vi "HOST_0505_2518.vi"() -> ()   [LabVIEW 2018]
uses:
  <vilib>/userdefined/High Color/nirio_resource_hc.ctl
  <instrlib>/niDCPower/nidcpower.llb/niDCPower Measurement Type.ctl
  <vilib>/FPGAPlugInAG/PXI-7953R/niLvFpga_Open_PXI-7953R.vi
  <vilib>/rvi/interface/common/dynamic/niFpgaDynamicAddResources.vi
  <vilib>/FPGAPlugInAG/Dynamic/niLvFpga_Reset_Dynamic.vi
  <vilib>/FPGAPlugInAG/Dynamic/niLvFpga_Run_Dynamic.vi
  <vilib>/Utility/error.llb/Error Cluster From Error Code.vi
  <vilib>/rvi/errors/niLvFpgaAdjustHostInterfaceError.vi
  <vilib>/FPGAPlugInAG/Dynamic/niLvFpga_Close_Dynamic.vi
  <vilib>/rvi/interface/nirviOpenFPGA/nirviOpenFPGA.xnode
  GSENSE2020BSI/FPGA Bitfiles/GSENSE2020_FPGATarget_Target_dmqGfihq6bQ.lvbitx
  <vilib>/rvi/interface/nirviMethod/nirviMethod.xnode
  <vilib>/rvi/interface/nirviReadWriteControl/nirviReadWriteControl.xnode
  <vilib>/rvi/interface/nirviCloseFPGA/nirviCloseFPGA.xnode
  NiFpgaLv.dll
  <vilib>/rvi/interface/Simulation/niFpgaSimulationCallBeginRW.vi
panel:
  out "SPI_OUT":bool[](array[boolean])
  in  "Запись":bool[](array[boolean])=[TRUE, TRUE, FALSE, FALSE, FALSE, FALSE, FALSE, FALSE, TRUE, FALSE, TRUE, FALSE, TRUE, TRUE, TRUE, FALSE, FALSE, TRUE, FALSE, FALSE, TRUE, TRUE, FALSE, FALSE, TRUE, TRUE, FALSE, TRUE, TRUE, TRUE, FALSE, FALSE, FALSE, TRUE, TRUE, FALSE, FALSE, TRUE, TRUE, TRUE, TRUE, FALSE, FALSE, TRUE, FALSE, TRUE, FALSE, FALSE, FALSE, TRUE, FALSE, TRUE, TRUE, FALSE, TRUE, TRUE, TRUE, TRUE, TRUE, FALSE, TRUE, TRUE, TRUE, FALSE, TRUE, FALSE, FALSE, FALSE, TRUE, TRUE, TRUE, FALSE, FALSE, FALSE, FALSE, FALSE, FALSE, FALSE, FALSE, FALSE, FALSE, FALSE, FALSE, FALSE, FALSE, FALSE, TRUE, TRUE, TRUE, TRUE, FALSE, FALSE, FALSE, FALSE, FALSE, TRUE, TRUE, FALSE, TRUE, FALSE, TRUE, FALSE, FALSE, FALSE, FALSE, TRUE, FALSE, FALSE, FALSE, TRUE, TRUE, FALSE, TRUE, FALSE, FALSE, FALSE, TRUE, TRUE, TRUE, TRUE, TRUE, FALSE, FALSE, TRUE, FALSE, FALSE, FALSE, TRUE, TRUE, FALSE, TRUE, FALSE, FALSE, TRUE, TRUE, TRUE, TRUE, TRUE, TRUE, FALSE, FALSE, TRUE, TRUE, FALSE, FALSE, TRUE, TRUE, TRUE, TRUE, FALSE, FALSE, TRUE, TRUE, FALSE, FALSE, FALSE, FALSE, FALSE, TRUE, TRUE, FALSE, FALSE, TRUE, FALSE, FALSE, FALSE, FALSE, FALSE, FALSE, FALSE, FALSE, FALSE, FALSE, FALSE, FALSE, FALSE, FALSE, FALSE, FALSE, FALSE, TRUE, FALSE, FALSE, FALSE, FALSE, FALSE, FALSE, FALSE, TRUE, TRUE, FALSE, TRUE, TRUE, TRUE, TRUE, FALSE, TRUE, FALSE, FALSE, FALSE, FALSE, FALSE, FALSE, FALSE, FALSE, FALSE, FALSE, TRUE, TRUE, TRUE, TRUE, TRUE, TRUE, TRUE, TRUE, FALSE, FALSE, TRUE, TRUE, FALSE, FALSE, TRUE, TRUE, TRUE, TRUE, TRUE, TRUE, TRUE, FALSE, FALSE, FALSE, FALSE, TRUE, TRUE, TRUE, FALSE, TRUE, TRUE, FALSE, TRUE, FALSE, TRUE, FALSE, FALSE, FALSE, FALSE, FALSE, FALSE, FALSE, TRUE, TRUE, TRUE, FALSE, TRUE, TRUE, FALSE]
  in  "3,3V_LVDS, V":dbl caption="voltage level" format="%_6p"
  in  "3,3V_LVDS_curlim":dbl=0.1 caption="current limit" format="%_6p"
  out "3,3V_LVDS_char":dbl(graph)=1.5967060684808935e-06
  in  "VDDPIX, V":dbl caption="voltage level" format="%_6p"
  in  "VDDPIX_curlim":dbl=0.1 caption="current limit" format="%_6p"
  out "VDDPIX_char":dbl(graph)=1.5967060684808935e-06
  in  "VG_RSTH, V":dbl caption="voltage level" format="%_6p"
  in  "VG_RSTH_curlim":dbl=0.1 caption="current limit" format="%_6p"
  out "VG_RSTH_char":dbl(graph)=1.5967060684808935e-06
  in  "LED, V":dbl caption="voltage level" format="%_6p"
  in  "LED_curlim":dbl=0.1 caption="current limit" format="%_6p"
  out "LED_char":dbl(graph)=1.5967060684808935e-06
  in  "VDD33A, V":dbl caption="voltage level" format="%_6p"
  in  "VDD33A_curlim":dbl=0.1 caption="current limit" format="%_6p"
  out "VDD33A_char":dbl(graph)=1.5967060684808935e-06
  in  "W(T)/R(F)":bool
  in  "Автомат":bool
  in  "VTXH, V":dbl caption="voltage level" format="%_6p"
  in  "VDDIO, V":dbl caption="voltage level" format="%_6p"
  in  "VDDCL, V":dbl caption="voltage level" format="%_6p"
  in  "VDD13, V":dbl caption="voltage level" format="%_6p"
  in  "VTXH_curlim":dbl=0.1 caption="current limit" format="%_6p"
  in  "VGRSTL_curlim":dbl=0.1 caption="current limit" format="%_6p"
  in  "VDDIO_curlim":dbl=0.1 caption="current limit" format="%_6p"
  in  "VDDCL_curlim":dbl=0.1 caption="current limit" format="%_6p"
  in  "VTXL_curlim":dbl=0.09 caption="current limit" format="%_6p"
  in  "VDD13_curlim":dbl=0.1 caption="current limit" format="%_6p"
  in  "VGRSTL, V":dbl caption="voltage level" format="%_6p"
  in  "VTXL, V":dbl caption="voltage level" format="%_6p"
  out "VTXH_char":dbl(graph)=-0.007753012065680951
  out "VGRSTL_char":dbl(graph)=6.909391540672134e-05
  out "VDDIO_char":dbl(graph)=9.424895165128459e-05
  out "VDDCL_char":dbl(graph)=-9.950040532110056e-06
  out "VTXL_char":dbl(graph)=9.067752968783287e-05
  out "VDD13_char":dbl(graph)=1.5967060684808935e-06
  in  "VDDPIX_selcur":dbl=0.09 caption="current limit" format="%_6p"
  in  "VDD33A_selcur":dbl=0.09 caption="current limit" format="%_6p"
  in  "VDD13_selcur":dbl=0.09 caption="current limit" format="%_6p"
  in  "VTXL_selcur":dbl=0.1 caption="current limit" format="%_6p"
  out "VDDCL_cur":dbl caption="measurement" format="%_6g"
  out "VTXL_cur":dbl caption="measurement" format="%_6g"
  out "VDD13_cur":dbl caption="measurement" format="%_6g"
  out "VDD33A_cur":dbl caption="measurement" format="%_6g"
  in  "SEL_Time, ms":u32=100
  in  "VG_RSTH_selcur":dbl=0.09 caption="current limit" format="%_6p"
  in  "VTXH_selcur":dbl=0.09 caption="current limit" format="%_6p"
  in  "VGRSTL_selcur":dbl=0.09 caption="current limit" format="%_6p"
  in  "VDDIO_selcur":dbl=0.09000000000000001 caption="current limit" format="%_6p"
  in  "VDDCL_selcur":dbl=0.09 caption="current limit" format="%_6p"
  out "VDDPIX_cur":dbl caption="measurement" format="%_6g"
  out "VDDIO_cur":dbl caption="measurement" format="%_6g"
  out "VGRSTL_cur":dbl caption="measurement" format="%_6g"
  out "VTXH_cur":dbl caption="measurement" format="%_6g"
  out "VG_RSTH_cur":dbl caption="measurement" format="%_6g"
  out "VDDPIX":u16
  out "VDDPIX":bool
  out "VDD33A":u16
  out "VDD33A":bool
  out "VDD13":u16
  out "VDD13":bool
  out "VTXL":u16
  out "VTXL":bool
  in  "3":refnum<k15>="PXI1Slot7" caption="1"
  in  "Проверка сбоев":bool
  out "SEU":bool
  out "SEU":u16
  in  "SPI":bool
  out "REG":bool
  in  "SAVE":bool
  in  "MOVIE":bool
  out "Картинка":bool
  out "Записали FIFO":bool
  in  "Хватит ждать!":bool
  in  "FRAME!":bool
  in  "SYS_RESET_N":bool
  out "SEL":bool
  in  "SIM_SEL":bool
  out "VG_RSTH":u16
  out "VDDCL":u16
  out "VTXH":u16
  out "VDDIO":u16
  out "VGRSTL":u16
  out "VG_RSTH":bool
  out "VDDCL":bool
  out "VTXH":bool
  out "VDDIO":bool
  out "VGRSTL":bool
  in  "Стоп":bool
  in  "Питание":bool
  in  "LED":bool caption="output enabled"
  in  "0":refnum<k15>="PXI1Slot5" caption="1"
  in  "1":refnum<k15>="PXI1Slot6"
  in  "2":refnum<k15>="PXI1Slot7" caption="1"
  in  "resource name 2":T1="PXI1Slot9"
  in  "SEU":path=path "C:/VPL/LabView/GSENSE2020BSI/SEU"
  in  "SEL":path=path "C:/VPL/LabView/GSENSE2020BSI/SEL"
  out "Номер образца":string="1"
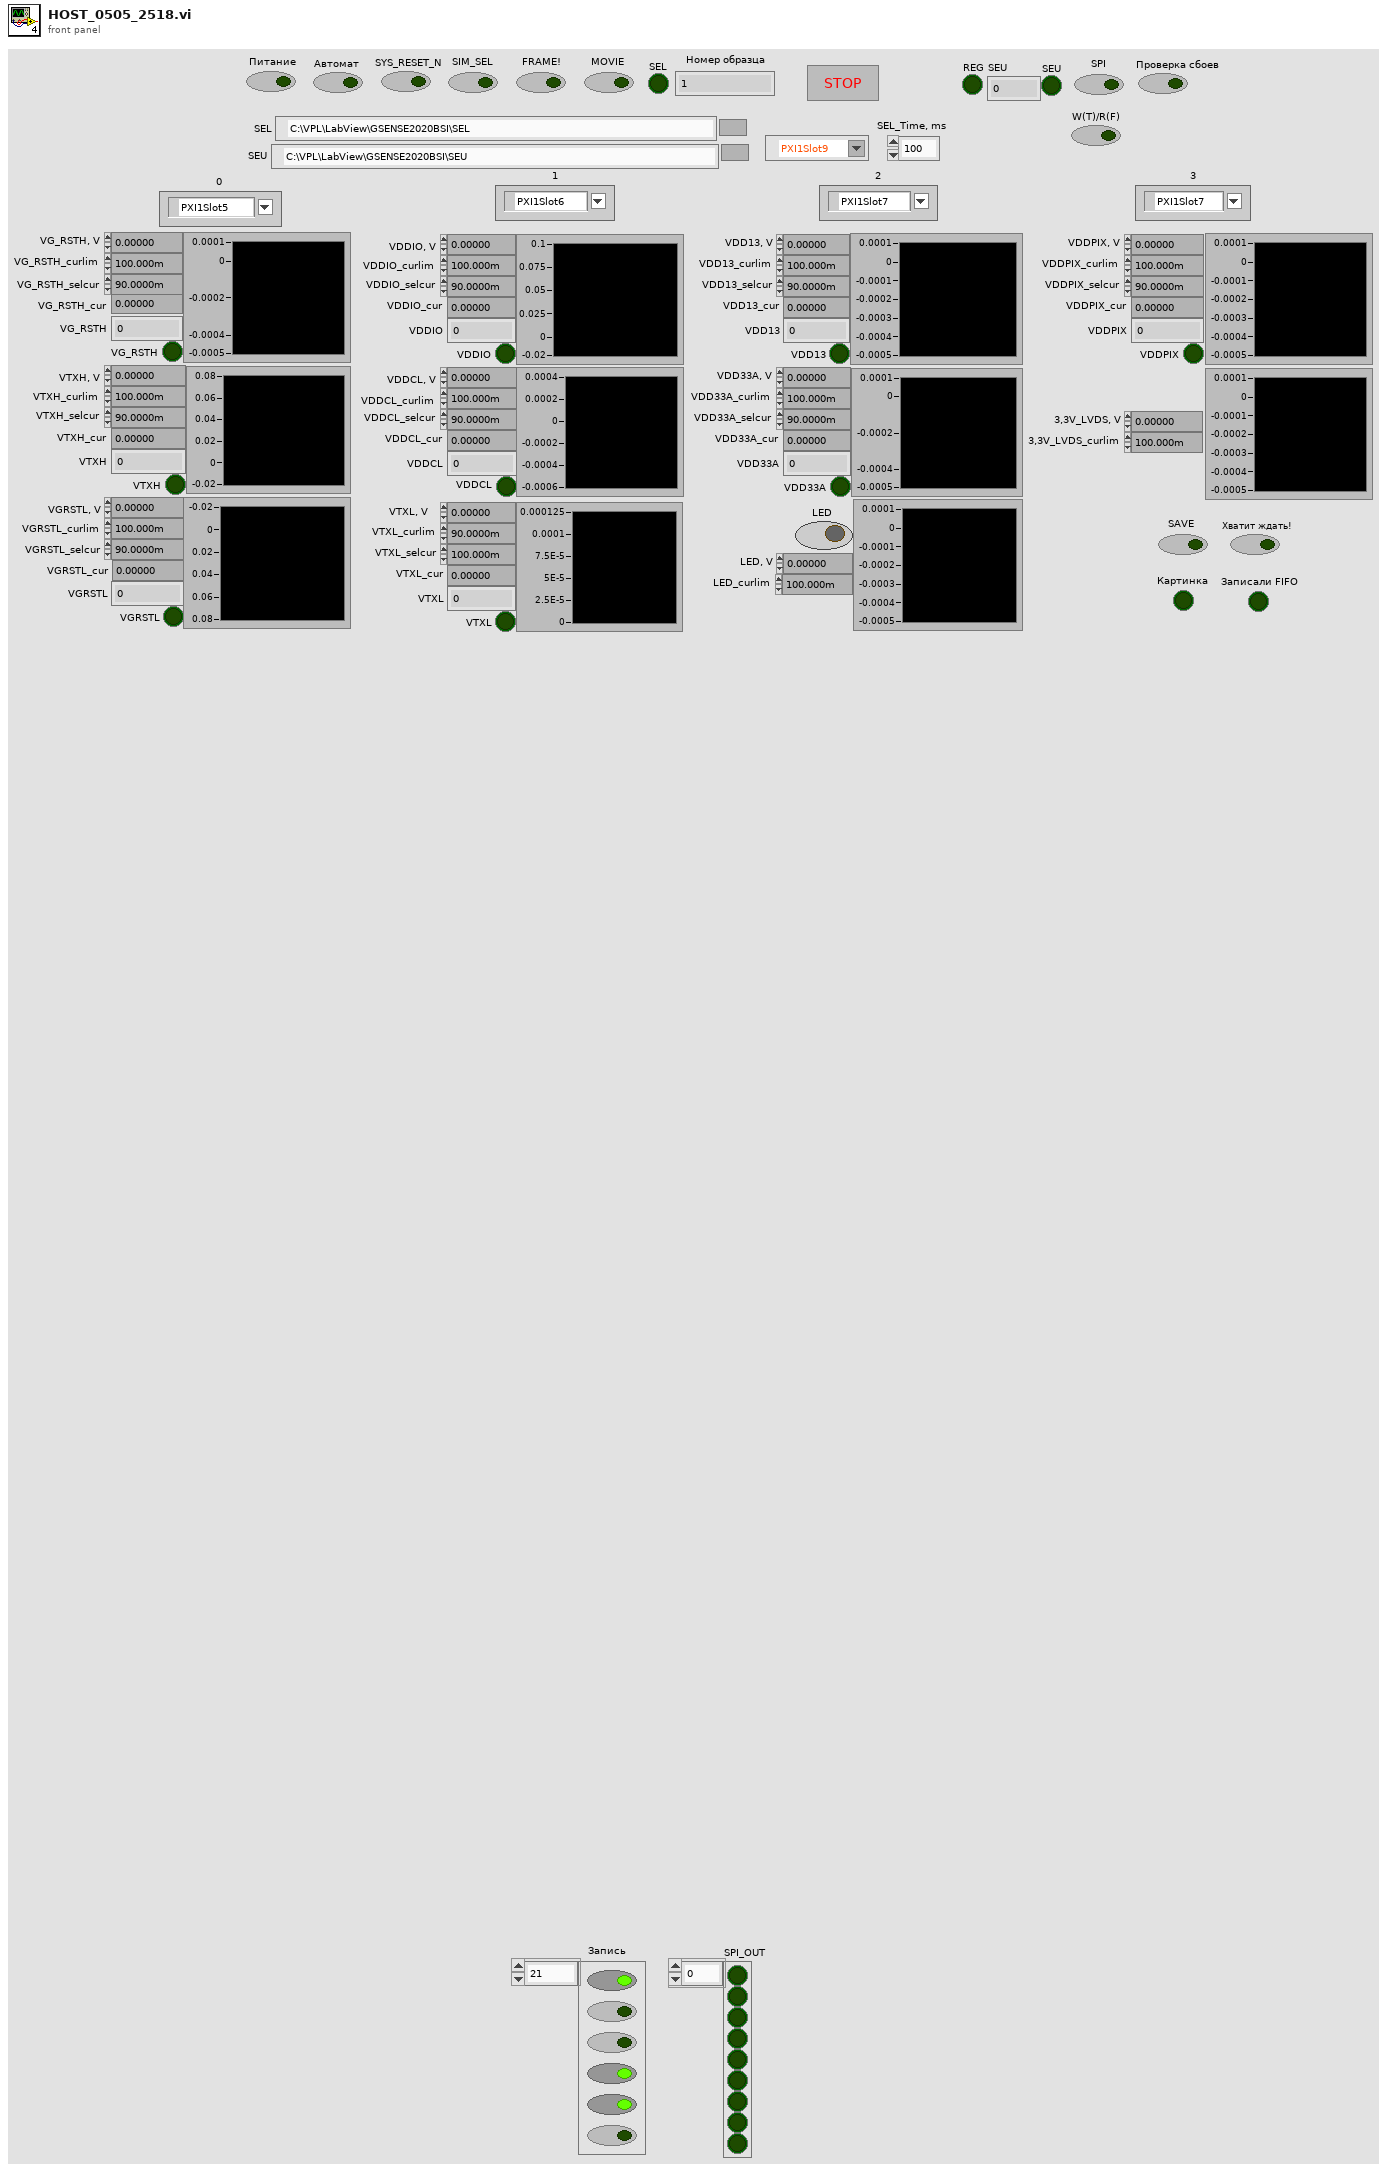
[diagram p1: front panel]
types:
  T1 = typedef "nirio_resource_hc.ctl" = tag
  T2 = enum16{"open", "replace", "create", "open or create", "replace or create", "replace or create with confirmation"}
  T3 = typedef "niDCPower Measurement Type.ctl" = i32
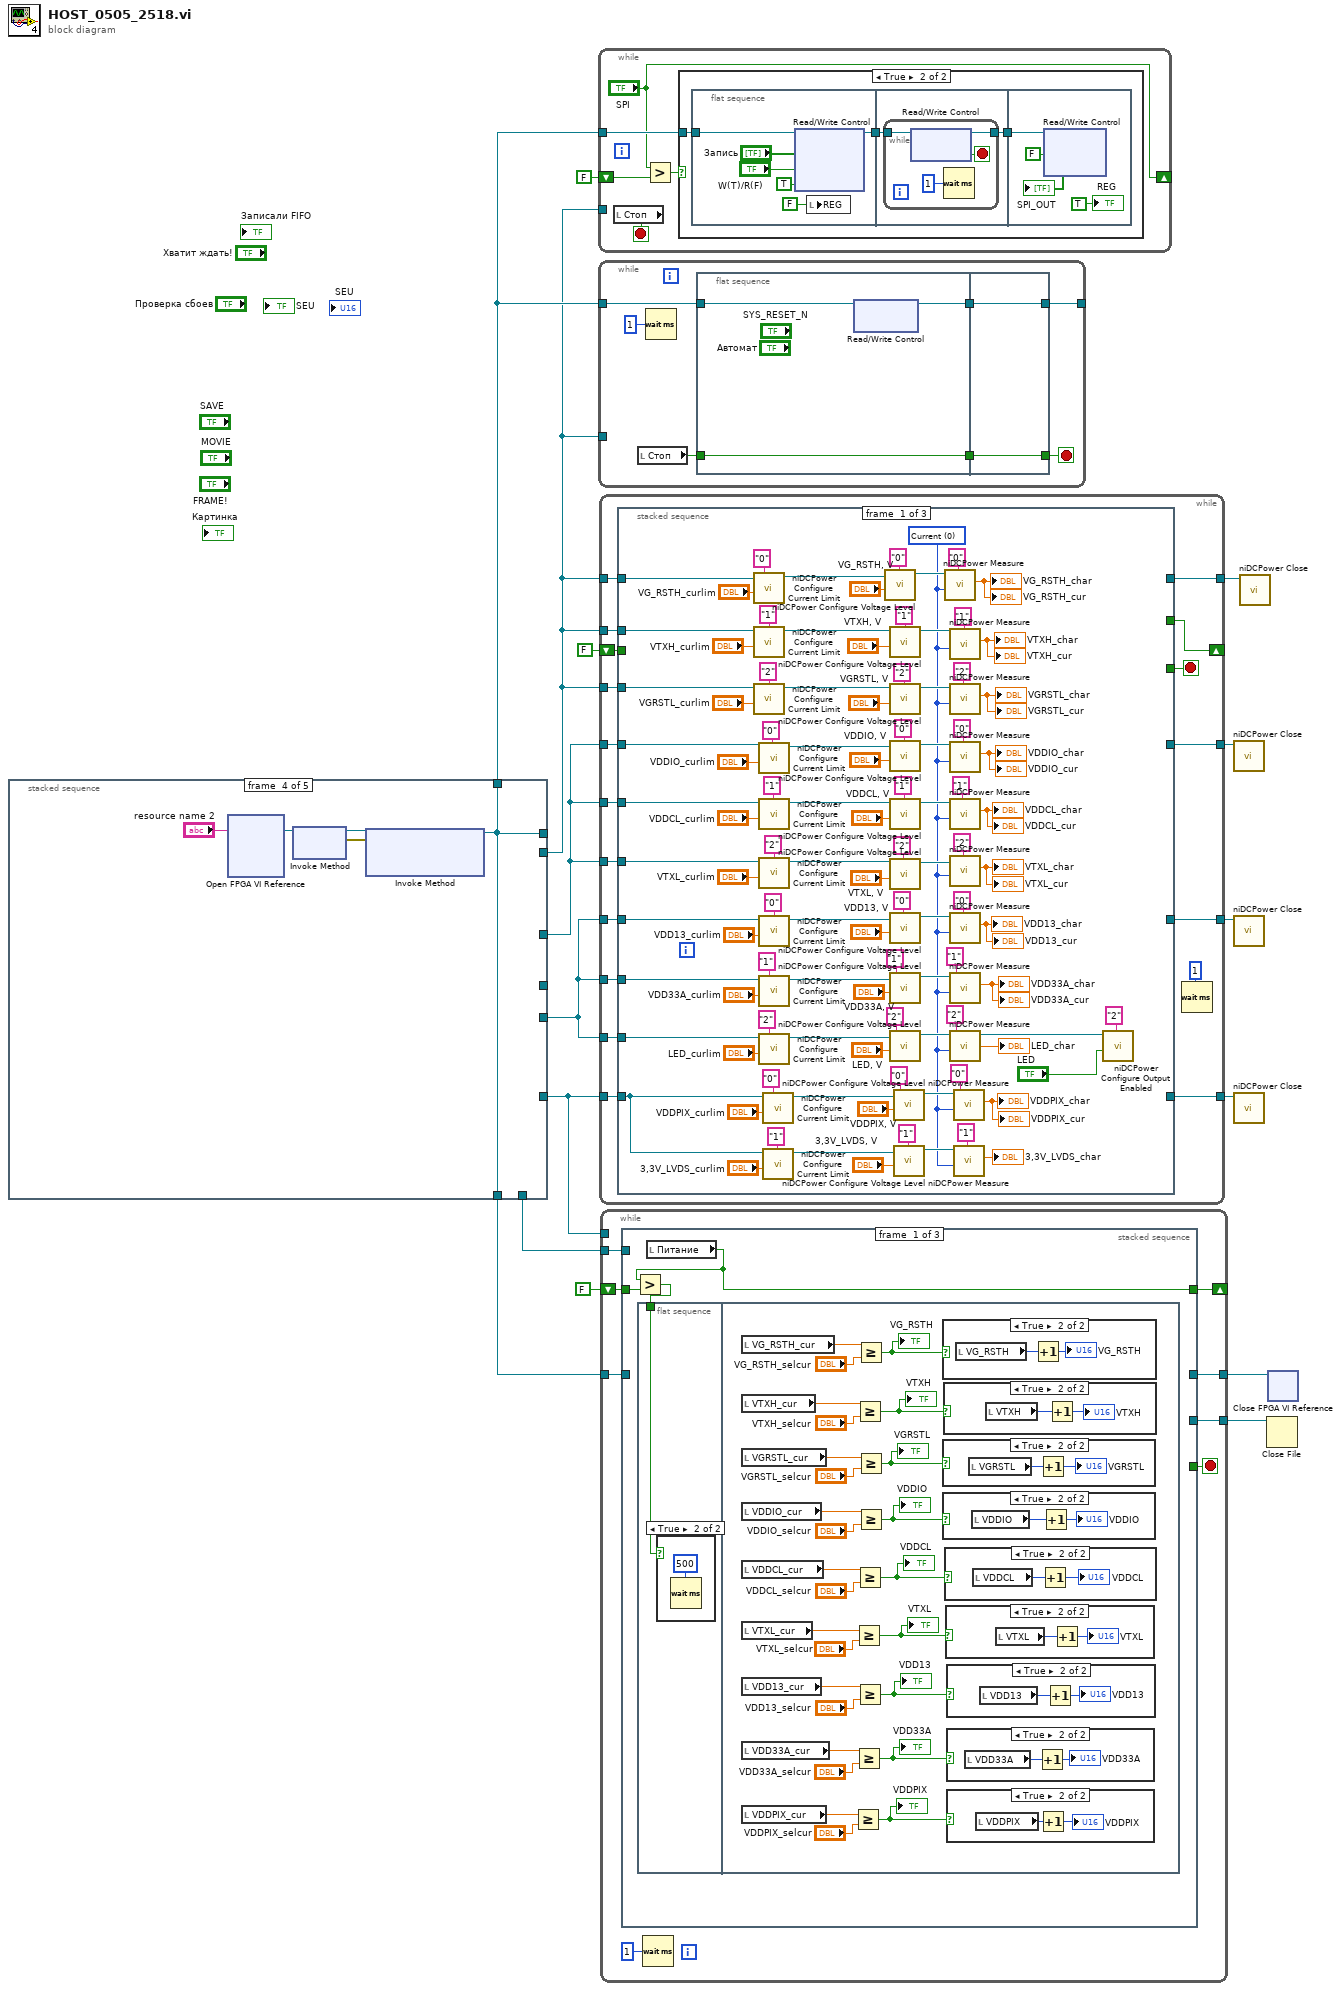
[diagram p0: block diagram]
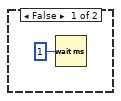
[diagram p2: hidden frame]
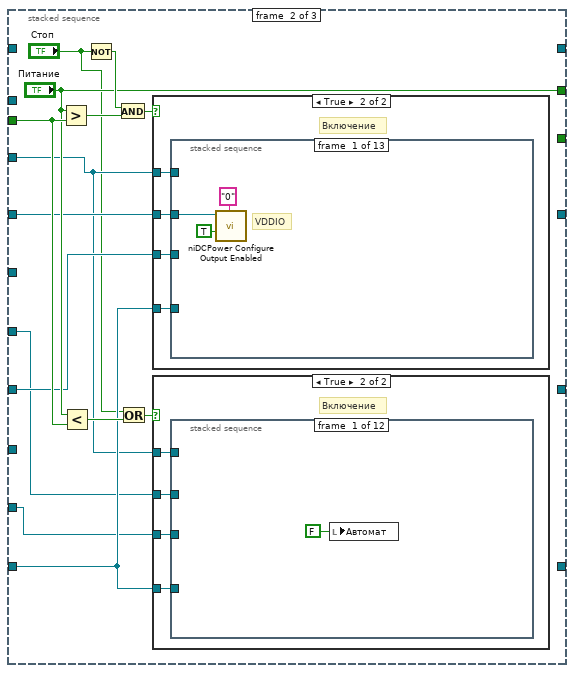
[diagram p3: hidden frame]
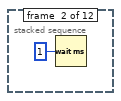
[diagram p5: hidden frame]
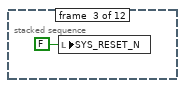
[diagram p6: hidden frame]
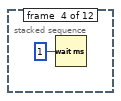
[diagram p7: hidden frame]
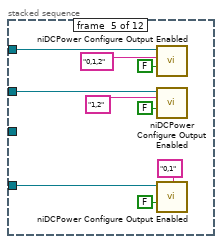
[diagram p8: hidden frame]
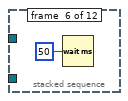
[diagram p9: hidden frame]
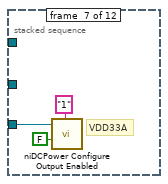
[diagram p10: hidden frame]
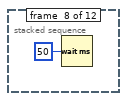
[diagram p11: hidden frame]
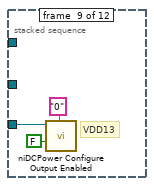
[diagram p12: hidden frame]
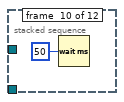
[diagram p13: hidden frame]
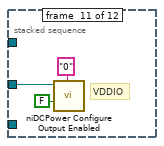
[diagram p14: hidden frame]
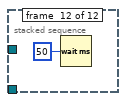
[diagram p15: hidden frame]
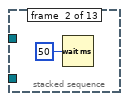
[diagram p17: hidden frame]
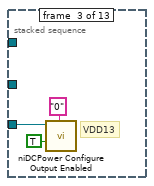
[diagram p18: hidden frame]
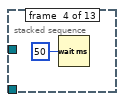
[diagram p19: hidden frame]
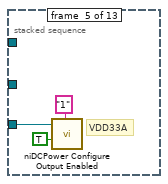
[diagram p20: hidden frame]
diagram:
  n1 = stacked-sequence {
    tunnel: [_ _ _ _ w101] -> w8
    tunnel: [_ _ _ _ w94] -> w1
    tunnel: [_ _ _ _ w105] -> w9
    tunnel: [_ _ _ w91 _] -> w2
    tunnel: [_ _ _ w91 _] -> w12
    tunnel: [_ w28 _ _ _] -> w13
    tunnel: [_ _ w58 _ _] -> _
    tunnel: [_ _ _ w91 _] -> _
    tunnel: [_ _ _ _ w95] -> w10
    frame #0 {
      w17 = FALSE ("Стоп")
      w19 = FALSE ("Стоп")
      w20 = u16 0 ("ADC")
      # "Обнуление"
      n2 = call "Begin.vi"() -> ("Номер образца 2"=→"Номер образца":string)  [unwired: 11 in]
      n3 = local write "VTXH"(w17) -> ()
      n4 = local write "SIM_SEL"(w17) -> ()
      n5 = local write "SPI"(w17) -> ()
      n6 = local write "Проверка сбоев"(w17) -> ()
      n7 = local write "SEL"(w17) -> ()
      n8 = local write "REG"(w17) -> ()
      n9 = local write "SEU"(w20) -> ()
      n10 = local write "VTXH"(w20) -> ()
      n11 = local write "VDDCL"(w20) -> ()
      n12 = local write "VG_RSTH"(w20) -> ()
      n13 = local write "VDDIO"(w20) -> ()
      n14 = local write "VGRSTL"(w20) -> ()
      n15 = local write "SYS_RESET_N"(w19) -> ()
      n16 = local write "SEU"(w19) -> ()
      n17 = local write "SAVE"(w19) -> ()
      n18 = local write "Хватит ждать!"(w19) -> ()
      n19 = local write "Записали FIFO"(w19) -> ()
      n20 = local write "Стоп"(w19) -> ()
      n21 = local write "Питание"(w19) -> ()
      n22 = local write "FRAME!"(w19) -> ()
      n23 = local write "MOVIE"(w19) -> ()
      n24 = local write "Картинка"(w19) -> ()
      n25 = local write "LED"(w19) -> ()
      n26 = local write "VG_RSTH"(w19) -> ()
      n27 = local write "VDDCL"(w19) -> ()
      n28 = local write "VGRSTL"(w19) -> ()
      n29 = local write "VDDIO"(w19) -> ()
    }
    frame #1 {
      w23 = "\t"
      # "Лог по токам"
      n30 = local read "Номер образца"() -> (w50:string)
      n31 = Build Path(base path="SEL", name or relative path=w50) -> (appended path=w47:path)
      n32 = Get Date/Time In Seconds() -> (seconds since 1Jan1904=w44:timestamp)
      n33 = call <vilib>:"Check if File or Folder Exists.vi"("path"=w47) -> ("file or folder exists?"=w48:bool, "dup path"=w49:path)  [unwired: 8 in, 1 out]
      n34 = Format Date/Time String(time format string (%c)="%d %H.%M.%S", seconds (now)=w44) -> (date/time string=w42:string)  [unwired: 1 in]
      n35 = case shown="False" w48 {
        tunnel: w49 -> [w56 w57]
        tunnel: [w55 w57] -> w22
        frame False {
          n36 = Create Folder(path (use dialog)=w56) -> (created path=w55:path)  [unwired: 2 in, 2 out]
        }
        frame True {
        }
      }
      n37 = Concatenate Strings(w42, ".xls" ("string")) -> (w41:string)
      n38 = Build Path(base path=w22, name or relative path=w41) -> (appended path=w43:path)
      n39 = Open/Create/Replace File(file path (use dialog)=w43, operation (0:open)=T2."open or create", access (0:read/write)=enum16{"read/write", "read-only", "write-only"}."read/write") -> (refnum out=w45:refnum<file>)  [unwired: 3 in, 2 out]
      n40 = case shown="True" TRUE {
        tunnel: w45 -> [w51 w54]
        tunnel: [w51 w52] -> w40
        frame False {
        }
        frame True {
          n41 = Set File Position(refnum=w54, from (0:start)=enum16{"start", "end", "current"}."end") -> (refnum out=w52:refnum<file>)  [unwired: 2 in, 1 out]
        }
      }
      n42 = Format Into String(initial string=w40, "Time" ("input 1"), w23, "VG_RSTH_cur", w23, "VTXH_cur", w23, "VGRSTL_cur", w23, "VDDIO_cur", w23, "VDDCL_cur", w23, "VTXL_cur", w23, "VDD13_cur", w23, "VDD33A_cur", w23, "VDDPIX_cur", w23, "\r\n") -> (resulting string=w28:refnum<file>)  [unwired: 2 in, 1 out]
    }
    frame #2 {
      w61 = "\t"
      # "Лог по сбоям"
      n43 = local read "Номер образца"() -> (w65:string)
      n44 = Build Path(base path="SEU", name or relative path=w65) -> (appended path=w79:path)
      n45 = Get Date/Time In Seconds() -> (seconds since 1Jan1904=w77:timestamp)
      n46 = call <vilib>:"Check if File or Folder Exists.vi"("path"=w79) -> ("file or folder exists?"=w80:bool, "dup path"=w81:path)  [unwired: 8 in, 1 out]
      n47 = Format Date/Time String(time format string (%c)="%d %H.%M.%S", seconds (now)=w77) -> (date/time string=w75:string)  [unwired: 1 in]
      n48 = case shown="False" w80 {
        tunnel: w81 -> [w87 w88]
        tunnel: [w86 w88] -> w66
        frame False {
          n49 = Create Folder(path (use dialog)=w87) -> (created path=w86:path)  [unwired: 2 in, 2 out]
        }
        frame True {
        }
      }
      n50 = Concatenate Strings(w75, ".xls" ("string")) -> (w74:string)
      n51 = Build Path(base path=w66, name or relative path=w74) -> (appended path=w76:path)
      n52 = Open/Create/Replace File(file path (use dialog)=w76, operation (0:open)=T2."open or create", access (0:read/write)=enum16{"read/write", "read-only", "write-only"}."read/write") -> (refnum out=w78:refnum<file>)  [unwired: 3 in, 2 out]
      n53 = case shown="True" TRUE {
        tunnel: w78 -> [w82 w85]
        tunnel: [w82 w83] -> w73
        frame False {
        }
        frame True {
          n54 = Set File Position(refnum=w85, from (0:start)=enum16{"start", "end", "current"}."end") -> (refnum out=w83:refnum<file>)  [unwired: 2 in, 1 out]
        }
      }
      n55 = Format Into String(initial string=w73, "Time" ("input 1"), w61, "Регистр №" ("input 3"), w61, "Содержание" ("input 4"), w61, "Кол-во сбоев" ("input 7"), "\r\n") -> (resulting string=w58:refnum<file>)  [unwired: 2 in, 1 out]
    }
    frame #3 {
      n56 = xnode "Open FPGA VI Reference"("resource name"="resource name 2") -> ("FPGA VI Reference Out"=w89:refnum<k20>)  [unwired: 1 in, 1 out]
      n57 = xnode "Invoke Method"("FPGA VI Reference In"=w89) -> ("FPGA VI Reference Out"=w93:refnum<k20>, "error out"=w92:errorcluster)  [unwired: 1 in]
      n58 = xnode "Invoke Method"("FPGA VI Reference In"=w93, "error in"=w92) -> ("FPGA VI Reference Out"=w91:refnum<k20>)  [unwired: 1 in, 1 out]
    }
    frame #4 {
      n59 = call <instrlib>:"niDCPower Initialize.vi"("resource name"="2") -> ("error out"=w111:errorcluster, "instrument handle out"=w108:refnum<k15>)  [unwired: 3 in, 6 out]
      n60 = call <instrlib>:"niDCPower Initialize.vi"("resource name"="1") -> ("error out"=w109:errorcluster, "instrument handle out"=w106:refnum<k15>)  [unwired: 3 in, 6 out]
      n61 = call <instrlib>:"niDCPower Initialize.vi"("resource name"="3") -> ("error out"=w99:errorcluster, "instrument handle out"=w100:refnum<k15>)  [unwired: 3 in, 6 out]
      n62 = call <instrlib>:"niDCPower Initialize.vi"("resource name"="0") -> ("error out"=w110:errorcluster, "instrument handle out"=w107:refnum<k15>)  [unwired: 3 in, 6 out]
      n63 = call <instrlib>:"niDCPower Configure Voltage Level.vi"("error in (no error)"=w111, "voltage level"=0.0, "channel name"="0,1,2", "instrument handle"=w108) -> ("instrument handle out"=w101:refnum<k15>)  [unwired: 6 in, 1 out]
      n64 = call <instrlib>:"niDCPower Configure Voltage Level.vi"("error in (no error)"=w109, "voltage level"=0.0, "channel name"="0,1,2", "instrument handle"=w106) -> ("instrument handle out"=w105:refnum<k15>)  [unwired: 6 in, 1 out]
      n65 = call <instrlib>:"niDCPower Configure Voltage Level.vi"("error in (no error)"=w99, "voltage level"=0.0, "channel name"="0,1", "instrument handle"=w100) -> ("instrument handle out"=w95:refnum<k15>)  [unwired: 6 in, 1 out]
      n66 = call <instrlib>:"niDCPower Configure Voltage Level.vi"("error in (no error)"=w110, "voltage level"=0.0, "channel name"="0,1,2", "instrument handle"=w107) -> ("instrument handle out"=w94:refnum<k15>)  [unwired: 6 in, 1 out]
    }
  }
  n67 = while {
    tunnel: w2 -> [w119]
    shift-right: ["SPI"] -> _
    shift-left: FALSE ("SPI") -> [w121]
    tunnel: w1 -> [_]
    stop <- w122 stop-if-true
    n68 = local read "Стоп"() -> (w122:bool)
    n69 = Greater?(x="SPI", y=w121) -> (0:w120:bool)
    n70 = case shown="True" w120 {
      tunnel: w119 -> [_ w126]
      frame False {
        n71 = Wait (ms)(milliseconds to wait=u32 1) -> ()  [unwired: 1 out]
      }
      frame True {
        n72 = flat-sequence {
          tunnel: w126 -> [w132]
          tunnel: [w129] -> w125
          tunnel: w125 -> [w134]
          tunnel: [w133] -> w124
          tunnel: w124 -> [w142]
          frame #0 {
            n73 = xnode "Read/Write Control"("FPGA VI Reference In"=w132, "SPI_IN"="Запись", "W(T)/R(F)"="W(T)/R(F)", "SPI"=TRUE) -> ("FPGA VI Reference Out"=w129:refnum<k20>)  [unwired: 1 in, 1 out]
            n74 = local write "REG"(FALSE ("REG")) -> ()
          }
          frame #1 {
            n75 = while {
              tunnel: w134 -> [w138]
              tunnel: [w135] -> w133
              stop <- w137 stop-if-true
              n76 = xnode "Read/Write Control"("FPGA VI Reference In"=w138) -> ("FPGA VI Reference Out"=w135:refnum<k20>, "SPI_OFF"=w137:bool)  [unwired: 1 in, 1 out]
              n77 = Wait (ms)(milliseconds to wait=u32 1) -> ()  [unwired: 1 out]
            }
          }
          frame #2 {
            n78 = xnode "Read/Write Control"("FPGA VI Reference In"=w142, "SPI"=FALSE) -> ("SPI_OUT"=→"SPI_OUT":bool[])  [unwired: 1 in, 2 out]
            "REG" <- TRUE ("REG")
          }
        }
      }
    }
  }
  n79 = while {
    tunnel: w2 -> [w148]
    tunnel: [w147] -> _
    tunnel: w1 -> [_]
    stop <- w143 stop-if-true
    n80 = local read "Стоп"() -> (w144:bool)
    n81 = Wait (ms)(milliseconds to wait=u32 1) -> ()  [unwired: 1 out]
    n82 = flat-sequence {
      tunnel: w148 -> [w152]
      tunnel: [w151] -> w146
      tunnel: [w150] -> w145
      tunnel: w144 -> [w150]
      tunnel: [w154] -> w147
      tunnel: w146 -> [w154]
      tunnel: w145 -> [w153]
      tunnel: [w153] -> w143
      frame #0 {
        n83 = xnode "Read/Write Control"("FPGA VI Reference In"=w152) -> ("FPGA VI Reference Out"=w151:refnum<k20>)  [unwired: 2 in, 1 out]
      }
      frame #1 {
      }
    }
  }
  n84 = while {
    shift-right: [w171] -> _
    shift-left: FALSE -> [w172]
    tunnel: w1 -> [w170]
    tunnel: w9 -> [w164]
    tunnel: w8 -> [w161]
    tunnel: w10 -> [w169]
    tunnel: w1 -> [w166]
    tunnel: w1 -> [w165]
    tunnel: w9 -> [w163]
    tunnel: w9 -> [w162]
    tunnel: w8 -> [w160]
    tunnel: w8 -> [w159]
    tunnel: [w158] -> w7
    tunnel: [w157] -> w6
    tunnel: [w156] -> w5
    tunnel: [w155] -> w4
    stop <- w168 stop-if-true
    n85 = stacked-sequence {
      tunnel: w172 -> [_ w288 _]
      tunnel: [_ "Питание" _] -> w171
      tunnel: w170 -> [w184 _ w352]
      tunnel: w169 -> [w173 w279 w349]
      tunnel: [_ _ w353] -> w168
      tunnel: w166 -> [w183 _ _]
      tunnel: w165 -> [w182 w276 _]
      tunnel: w164 -> [w181 w282 w351]
      tunnel: w163 -> [w180 _ _]
      tunnel: w162 -> [w179 w277 _]
      tunnel: w161 -> [w178 w281 w350]
      tunnel: w160 -> [w177 _ _]
      tunnel: w159 -> [w176 w278 _]
      tunnel: [_ _ w352] -> w158
      tunnel: [_ _ w351] -> w157
      tunnel: [_ _ w350] -> w156
      tunnel: [_ _ w349] -> w155
      frame #0 {
        w198 = T3 0 items=["Current", "Voltage"] ("measurement type")
        n86 = call <instrlib>:"niDCPower Configure Current Limit.vi"("current limit"="VG_RSTH_curlim", "channel name"="0", "instrument handle"=w184) -> ("instrument handle out"=w215:refnum<k15>)  [unwired: 7 in, 1 out]
        n87 = call <instrlib>:"niDCPower Configure Current Limit.vi"("current limit"="VTXH_curlim", "channel name"="1", "instrument handle"=w183) -> ("instrument handle out"=w255:refnum<k15>)  [unwired: 7 in, 1 out]
        n88 = call <instrlib>:"niDCPower Configure Current Limit.vi"("current limit"="VGRSTL_curlim", "channel name"="2", "instrument handle"=w182) -> ("instrument handle out"=w256:refnum<k15>)  [unwired: 7 in, 1 out]
        n89 = call <instrlib>:"niDCPower Configure Current Limit.vi"("current limit"="VDDIO_curlim", "channel name"="0", "instrument handle"=w181) -> ("instrument handle out"=w257:refnum<k15>)  [unwired: 7 in, 1 out]
        n90 = call <instrlib>:"niDCPower Configure Current Limit.vi"("current limit"="VDDCL_curlim", "channel name"="1", "instrument handle"=w180) -> ("instrument handle out"=w258:refnum<k15>)  [unwired: 7 in, 1 out]
        n91 = call <instrlib>:"niDCPower Configure Current Limit.vi"("current limit"="VTXL_curlim", "channel name"="2", "instrument handle"=w179) -> ("instrument handle out"=w259:refnum<k15>)  [unwired: 7 in, 1 out]
        n92 = call <instrlib>:"niDCPower Configure Current Limit.vi"("current limit"="VDD13_curlim", "channel name"="0", "instrument handle"=w178) -> ("instrument handle out"=w260:refnum<k15>)  [unwired: 7 in, 1 out]
        n93 = call <instrlib>:"niDCPower Configure Current Limit.vi"("current limit"="VDD33A_curlim", "channel name"="1", "instrument handle"=w177) -> ("instrument handle out"=w228:refnum<k15>)  [unwired: 7 in, 1 out]
        n94 = call <instrlib>:"niDCPower Configure Current Limit.vi"("current limit"="LED_curlim", "channel name"="2", "instrument handle"=w176) -> ("instrument handle out"=w223:refnum<k15>)  [unwired: 7 in, 1 out]
        n95 = call <instrlib>:"niDCPower Configure Current Limit.vi"("current limit"="VDDPIX_curlim", "channel name"="0", "instrument handle"=w173) -> ("instrument handle out"=w208:refnum<k15>)  [unwired: 7 in, 1 out]
        n96 = call <instrlib>:"niDCPower Configure Current Limit.vi"("current limit"="3,3V_LVDS_curlim", "channel name"="1", "instrument handle"=w173) -> ("instrument handle out"=w203:refnum<k15>)  [unwired: 7 in, 1 out]
        n97 = call <instrlib>:"niDCPower Configure Voltage Level.vi"("voltage level"="VG_RSTH, V", "channel name"="0", "instrument handle"=w215) -> ("instrument handle out"=w218:refnum<k15>)  [unwired: 7 in, 1 out]
        n98 = call <instrlib>:"niDCPower Configure Voltage Level.vi"("voltage level"="VTXH, V", "channel name"="1", "instrument handle"=w255) -> ("instrument handle out"=w238:refnum<k15>)  [unwired: 7 in, 1 out]
        n99 = call <instrlib>:"niDCPower Configure Voltage Level.vi"("voltage level"="VGRSTL, V", "channel name"="2", "instrument handle"=w256) -> ("instrument handle out"=w237:refnum<k15>)  [unwired: 7 in, 1 out]
        n100 = call <instrlib>:"niDCPower Configure Voltage Level.vi"("voltage level"="VDDIO, V", "channel name"="0", "instrument handle"=w257) -> ("instrument handle out"=w236:refnum<k15>)  [unwired: 7 in, 1 out]
        n101 = call <instrlib>:"niDCPower Configure Voltage Level.vi"("voltage level"="VDDCL, V", "channel name"="1", "instrument handle"=w258) -> ("instrument handle out"=w235:refnum<k15>)  [unwired: 7 in, 1 out]
        n102 = call <instrlib>:"niDCPower Configure Voltage Level.vi"("voltage level"="VTXL, V", "channel name"="2", "instrument handle"=w259) -> ("instrument handle out"=w234:refnum<k15>)  [unwired: 7 in, 1 out]
        n103 = call <instrlib>:"niDCPower Configure Voltage Level.vi"("voltage level"="VDD13, V", "channel name"="0", "instrument handle"=w260) -> ("instrument handle out"=w233:refnum<k15>)  [unwired: 7 in, 1 out]
        n104 = call <instrlib>:"niDCPower Configure Voltage Level.vi"("voltage level"="VDD33A, V", "channel name"="1", "instrument handle"=w228) -> ("instrument handle out"=w231:refnum<k15>)  [unwired: 7 in, 1 out]
        n105 = call <instrlib>:"niDCPower Configure Voltage Level.vi"("voltage level"="LED, V", "channel name"="2", "instrument handle"=w223) -> ("instrument handle out"=w220:refnum<k15>)  [unwired: 7 in, 1 out]
        n106 = call <instrlib>:"niDCPower Configure Voltage Level.vi"("voltage level"="VDDPIX, V", "channel name"="0", "instrument handle"=w208) -> ("instrument handle out"=w211:refnum<k15>)  [unwired: 7 in, 1 out]
        n107 = call <instrlib>:"niDCPower Configure Voltage Level.vi"("voltage level"="3,3V_LVDS, V", "channel name"="1", "instrument handle"=w203) -> ("instrument handle out"=w200:refnum<k15>)  [unwired: 7 in, 1 out]
        n108 = call <instrlib>:"niDCPower Measure.vi"("measurement type"=w198, "channel name"="0", "instrument handle"=w218) -> ("measurement"=→"VG_RSTH_char" →"VG_RSTH_cur":dbl)  [unwired: 6 in, 2 out]
        n109 = call <instrlib>:"niDCPower Measure.vi"("measurement type"=w198, "channel name"="1", "instrument handle"=w238) -> ("measurement"=→"VTXH_char" →"VTXH_cur":dbl)  [unwired: 6 in, 2 out]
        n110 = call <instrlib>:"niDCPower Measure.vi"("measurement type"=w198, "channel name"="2", "instrument handle"=w237) -> ("measurement"=→"VGRSTL_char" →"VGRSTL_cur":dbl)  [unwired: 6 in, 2 out]
        n111 = call <instrlib>:"niDCPower Measure.vi"("measurement type"=w198, "channel name"="0", "instrument handle"=w236) -> ("measurement"=→"VDDIO_char" →"VDDIO_cur":dbl)  [unwired: 6 in, 2 out]
        n112 = call <instrlib>:"niDCPower Measure.vi"("measurement type"=w198, "channel name"="1", "instrument handle"=w235) -> ("measurement"=→"VDDCL_char" →"VDDCL_cur":dbl)  [unwired: 6 in, 2 out]
        n113 = call <instrlib>:"niDCPower Measure.vi"("measurement type"=w198, "channel name"="2", "instrument handle"=w234) -> ("measurement"=→"VTXL_char" →"VTXL_cur":dbl)  [unwired: 6 in, 2 out]
        n114 = call <instrlib>:"niDCPower Measure.vi"("measurement type"=w198, "channel name"="0", "instrument handle"=w233) -> ("measurement"=→"VDD13_char" →"VDD13_cur":dbl)  [unwired: 6 in, 2 out]
        n115 = call <instrlib>:"niDCPower Measure.vi"("measurement type"=w198, "channel name"="1", "instrument handle"=w231) -> ("measurement"=→"VDD33A_char" →"VDD33A_cur":dbl)  [unwired: 6 in, 2 out]
        n116 = call <instrlib>:"niDCPower Measure.vi"("measurement type"=w198, "channel name"="2", "instrument handle"=w220) -> ("measurement"=→"LED_char":dbl, "instrument handle out"=w186:refnum<k15>)  [unwired: 6 in, 1 out]
        n117 = call <instrlib>:"niDCPower Measure.vi"("measurement type"=w198, "channel name"="0", "instrument handle"=w211) -> ("measurement"=→"VDDPIX_char" →"VDDPIX_cur":dbl)  [unwired: 6 in, 2 out]
        n118 = call <instrlib>:"niDCPower Measure.vi"("measurement type"=w198, "channel name"="1", "instrument handle"=w200) -> ("measurement"=→"3,3V_LVDS_char":dbl)  [unwired: 6 in, 2 out]
        n119 = call <instrlib>:"niDCPower Configure Output Enabled.vi"("output enabled"="LED", "channel name"="2", "instrument handle"=w186) -> ()  [unwired: 7 in, 2 out]
      }
      frame #1 {
        n120 = Greater?(x="Питание", y=w288) -> (0:w286:bool)
        n121 = Less?(x="Питание", y=w288) -> (x < y?=w284:bool)
        n122 = Not(x="Стоп") -> (.not. x?=w285:bool)
        n123 = And(x=w285, y=w286) -> (x .and. y?=w287:bool)
        n124 = Or(x="Стоп", y=w284) -> (x .or. y?=w280:bool)
        n125 = case shown="True" w287 {
          tunnel: w282 -> [_ w322]
          tunnel: w281 -> [_ w321]
          tunnel: w276 -> [_ w320]
          tunnel: w279 -> [_ w319]
          frame False {
          }
          frame True {
            # "Включение"
            n126 = stacked-sequence {
              tunnel: w322 -> [w323 _ _ _ _ _ w339 _ _ _ _ _ _]
              tunnel: w321 -> [_ _ w327 _ w331 _ _ _ _ _ _ _ _]
              tunnel: w320 -> [_ _ _ _ _ _ w342 _ _ _ _ _ _]
              tunnel: w319 -> [_ _ _ _ _ _ w338 _ _ _ _ _ _]
              frame #0 {
                # "VDDIO"
                n127 = call <instrlib>:"niDCPower Configure Output Enabled.vi"("output enabled"=TRUE, "channel name"="0", "instrument handle"=w323) -> ()  [unwired: 7 in, 2 out]
              }
              frame #1 {
                n128 = Wait (ms)(milliseconds to wait=u32 50) -> ()  [unwired: 1 out]
              }
              frame #2 {
                # "VDD13"
                n129 = call <instrlib>:"niDCPower Configure Output Enabled.vi"("output enabled"=TRUE, "channel name"="0", "instrument handle"=w327) -> ()  [unwired: 7 in, 2 out]
              }
              frame #3 {
                n130 = Wait (ms)(milliseconds to wait=u32 50) -> ()  [unwired: 1 out]
              }
              frame #4 {
                # "VDD33А"
                n131 = call <instrlib>:"niDCPower Configure Output Enabled.vi"("output enabled"=TRUE, "channel name"="1", "instrument handle"=w331) -> ()  [unwired: 7 in, 2 out]
              }
              frame #5 {
                n132 = Wait (ms)(milliseconds to wait=u32 50) -> ()  [unwired: 1 out]
              }
              frame #6 {
                n133 = call <instrlib>:"niDCPower Configure Output Enabled.vi"("output enabled"=TRUE, "channel name"="0,1,2", "instrument handle"=w342) -> ()  [unwired: 7 in, 2 out]
                n134 = call <instrlib>:"niDCPower Configure Output Enabled.vi"("output enabled"=TRUE, "channel name"="1,2", "instrument handle"=w339) -> ()  [unwired: 7 in, 2 out]
                n135 = call <instrlib>:"niDCPower Configure Output Enabled.vi"("output enabled"=TRUE, "channel name"="0,1", "instrument handle"=w338) -> ()  [unwired: 7 in, 2 out]
              }
              frame #7 {
                n136 = Wait (ms)(milliseconds to wait=u32 50) -> ()  [unwired: 1 out]
              }
              frame #8 {
                n137 = local write "SYS_RESET_N"(TRUE ("SYS_RESET_N")) -> ()
              }
              frame #9 {
                n138 = Wait (ms)(milliseconds to wait=u32 1) -> ()  [unwired: 1 out]
              }
              frame #10 {
                n139 = local write "Автомат"(TRUE ("Автомат")) -> ()
              }
              frame #11 {
                n140 = Wait (ms)(milliseconds to wait=u32 1) -> ()  [unwired: 1 out]
              }
              frame #12 {
                # "Прошиваем регистры"
              }
            }
          }
        }
        n141 = case shown="True" w280 {
          tunnel: w277 -> [_ w292]
          tunnel: w278 -> [_ w291]
          tunnel: w276 -> [_ w290]
          tunnel: w279 -> [_ w289]
          frame False {
          }
          frame True {
            # "Включение"
            n142 = stacked-sequence {
              tunnel: w292 -> [_ _ _ _ w301 _ _ _ _ _ w315 _]
              tunnel: w291 -> [_ _ _ _ _ _ w307 _ w311 _ _ _]
              tunnel: w290 -> [_ _ _ _ w304 _ _ _ _ _ _ _]
              tunnel: w289 -> [_ _ _ _ w300 _ _ _ _ _ _ _]
              frame #0 {
                n143 = local write "Автомат"(FALSE ("Автомат")) -> ()
              }
              frame #1 {
                n144 = Wait (ms)(milliseconds to wait=u32 1) -> ()  [unwired: 1 out]
              }
              frame #2 {
                n145 = local write "SYS_RESET_N"(FALSE ("SYS_RESET_N")) -> ()
              }
              frame #3 {
                n146 = Wait (ms)(milliseconds to wait=u32 1) -> ()  [unwired: 1 out]
              }
              frame #4 {
                n147 = call <instrlib>:"niDCPower Configure Output Enabled.vi"("output enabled"=FALSE, "channel name"="0,1,2", "instrument handle"=w304) -> ()  [unwired: 7 in, 2 out]
                n148 = call <instrlib>:"niDCPower Configure Output Enabled.vi"("output enabled"=FALSE, "channel name"="1,2", "instrument handle"=w301) -> ()  [unwired: 7 in, 2 out]
                n149 = call <instrlib>:"niDCPower Configure Output Enabled.vi"("output enabled"=FALSE, "channel name"="0,1", "instrument handle"=w300) -> ()  [unwired: 7 in, 2 out]
              }
              frame #5 {
                n150 = Wait (ms)(milliseconds to wait=u32 50) -> ()  [unwired: 1 out]
              }
              frame #6 {
                # "VDD33А"
                n151 = call <instrlib>:"niDCPower Configure Output Enabled.vi"("output enabled"=FALSE, "channel name"="1", "instrument handle"=w307) -> ()  [unwired: 7 in, 2 out]
              }
              frame #7 {
                n152 = Wait (ms)(milliseconds to wait=u32 50) -> ()  [unwired: 1 out]
              }
              frame #8 {
                # "VDD13"
                n153 = call <instrlib>:"niDCPower Configure Output Enabled.vi"("output enabled"=FALSE, "channel name"="0", "instrument handle"=w311) -> ()  [unwired: 7 in, 2 out]
              }
              frame #9 {
                n154 = Wait (ms)(milliseconds to wait=u32 50) -> ()  [unwired: 1 out]
              }
              frame #10 {
                # "VDDIO"
                n155 = call <instrlib>:"niDCPower Configure Output Enabled.vi"("output enabled"=FALSE, "channel name"="0", "instrument handle"=w315) -> ()  [unwired: 7 in, 2 out]
              }
              frame #11 {
                n156 = Wait (ms)(milliseconds to wait=u32 50) -> ()  [unwired: 1 out]
              }
            }
          }
        }
      }
      frame #2 {
        n157 = local read "Стоп"() -> (w353:bool)
      }
    }
    n158 = Wait (ms)(milliseconds to wait=u32 1) -> ()  [unwired: 1 out]
  }
  n159 = while {
    tunnel: w12 -> [w356]
    shift-right: [w360] -> _
    shift-left: FALSE ("Питание") -> [w361]
    tunnel: w13 -> [w358]
    tunnel: [w355] -> w15
    tunnel: [w354] -> w14
    tunnel: w10 -> [_]
    stop <- w357 stop-if-true
    n160 = stacked-sequence {
      tunnel: w361 -> [w364 _ _]
      tunnel: [w363 _ _] -> w360
      tunnel: w358 -> [_ w465 _]
      tunnel: [_ _ w485] -> w357
      tunnel: w356 -> [_ _ w484]
      tunnel: [_ w454 _] -> w355
      tunnel: [_ _ w482] -> w354
      frame #0 {
        n161 = flat-sequence {
          tunnel: w362 -> [w365]
          frame #0 {
            n162 = case shown="True" w365 {
              frame False {
              }
              frame True {
                n163 = Wait (ms)(milliseconds to wait=u32 500) -> ()  [unwired: 1 out]
              }
            }
          }
          frame #1 {
            n164 = local read "VG_RSTH_cur"() -> (w386:dbl)
            n165 = local read "VTXH_cur"() -> (w387:dbl)
            n166 = local read "VGRSTL_cur"() -> (w388:dbl)
            n167 = local read "VDDIO_cur"() -> (w389:dbl)
            n168 = local read "VDDCL_cur"() -> (w380:dbl)
            n169 = local read "VTXL_cur"() -> (w379:dbl)
            n170 = local read "VDD13_cur"() -> (w378:dbl)
            n171 = local read "VDD33A_cur"() -> (w377:dbl)
            n172 = local read "VDDPIX_cur"() -> (w376:dbl)
            n173 = Greater Or Equal?(x=w376, y="VDDPIX_selcur") -> (x >= y?=w367:bool)
            "VDDPIX" <- w367
            n174 = Greater Or Equal?(x=w379, y="VTXL_selcur") -> (x >= y?=w370:bool)
            "VTXL" <- w370
            n175 = Greater Or Equal?(x=w377, y="VDD33A_selcur") -> (x >= y?=w368:bool)
            "VDD33A" <- w368
            n176 = Greater Or Equal?(x=w387, y="VTXH_selcur") -> (x >= y?=w374:bool)
            "VTXH" <- w374
            n177 = Greater Or Equal?(x=w380, y="VDDCL_selcur") -> (x >= y?=w371:bool)
            "VDDCL" <- w371
            n178 = Greater Or Equal?(x=w378, y="VDD13_selcur") -> (x >= y?=w369:bool)
            "VDD13" <- w369
            n179 = Greater Or Equal?(x=w386, y="VG_RSTH_selcur") -> (x >= y?=w375:bool)
            "VG_RSTH" <- w375
            n180 = Greater Or Equal?(x=w388, y="VGRSTL_selcur") -> (x >= y?=w373:bool)
            "VGRSTL" <- w373
            n181 = Greater Or Equal?(x=w389, y="VDDIO_selcur") -> (x >= y?=w372:bool)
            "VDDIO" <- w372
            n182 = case shown="True" w375 {
              frame False {
              }
              frame True {
                n183 = local read "VG_RSTH"() -> (w410:u16)
                n184 = Increment(x=w410) -> (x+1=→"VG_RSTH":u16)
              }
            }
            n185 = case shown="True" w373 {
              frame False {
              }
              frame True {
                n186 = local read "VGRSTL"() -> (w406:u16)
                n187 = Increment(x=w406) -> (x+1=→"VGRSTL":u16)
              }
            }
            n188 = case shown="True" w372 {
              frame False {
              }
              frame True {
                n189 = local read "VDDIO"() -> (w404:u16)
                n190 = Increment(x=w404) -> (x+1=→"VDDIO":u16)
              }
            }
            n191 = case shown="True" w374 {
              frame False {
              }
              frame True {
                n192 = local read "VTXH"() -> (w408:u16)
                n193 = Increment(x=w408) -> (x+1=→"VTXH":u16)
              }
            }
            n194 = case shown="True" w371 {
              frame False {
              }
              frame True {
                n195 = local read "VDDCL"() -> (w402:u16)
                n196 = Increment(x=w402) -> (x+1=→"VDDCL":u16)
              }
            }
            n197 = case shown="True" w370 {
              frame False {
              }
              frame True {
                n198 = local read "VTXL"() -> (w400:u16)
                n199 = Increment(x=w400) -> (x+1=→"VTXL":u16)
              }
            }
            n200 = case shown="True" w369 {
              frame False {
              }
              frame True {
                n201 = local read "VDD13"() -> (w398:u16)
                n202 = Increment(x=w398) -> (x+1=→"VDD13":u16)
              }
            }
            n203 = case shown="True" w368 {
              frame False {
              }
              frame True {
                n204 = local read "VDD33A"() -> (w396:u16)
                n205 = Increment(x=w396) -> (x+1=→"VDD33A":u16)
              }
            }
            n206 = case shown="True" w367 {
              frame False {
              }
              frame True {
                n207 = local read "VDDPIX"() -> (w394:u16)
                n208 = Increment(x=w394) -> (x+1=→"VDDPIX":u16)
              }
            }
          }
        }
        n209 = local read "Питание"() -> (w363:bool)
        n210 = Greater?(x=w363, y=w364) -> (0:w362:bool)
      }
      frame #1 {
        w436 = "\t"
        w452 = i16 0 ("width (-)")
        w453 = i16 3 ("width (-)")
        n211 = local read "VG_RSTH_cur"() -> (w464:dbl)
        n212 = local read "VTXH_cur"() -> (w463:dbl)
        n213 = local read "VGRSTL_cur"() -> (w455:dbl)
        n214 = local read "VDDIO_cur"() -> (w451:dbl)
        n215 = local read "VDDCL_cur"() -> (w450:dbl)
        n216 = local read "VTXL_cur"() -> (w449:dbl)
        n217 = local read "VDD13_cur"() -> (w448:dbl)
        n218 = local read "VDD33A_cur"() -> (w447:dbl)
        n219 = local read "VDDPIX_cur"() -> (w446:dbl)
        n220 = local read "VG_RSTH"() -> (w445:u16)
        n221 = local read "VTXH"() -> (w444:u16)
        n222 = local read "VGRSTL"() -> (w443:u16)
        n223 = local read "VDDIO"() -> (w442:u16)
        n224 = local read "VDDCL"() -> (w441:u16)
        n225 = local read "VTXL"() -> (w440:u16)
        n226 = local read "VDD13"() -> (w439:u16)
        n227 = local read "VDD33A"() -> (w438:u16)
        n228 = local read "VDDPIX"() -> (w437:u16)
        n229 = Get Date/Time In Seconds() -> (seconds since 1Jan1904=w470:timestamp)
        n230 = Format Date/Time String(time format string (%c)="%d %H:%M:%S:%3u", seconds (now)=w470) -> (date/time string=w462:string)  [unwired: 1 in]
        n231 = Number To Fractional String(number=w464, width (-)=w453, precision (6)=w453) -> (F-format string=w461:string)  [unwired: 1 in]
        n232 = Number To Fractional String(number=w463, width (-)=w453, precision (6)=w453) -> (F-format string=w460:string)  [unwired: 1 in]
        n233 = Number To Fractional String(number=w455, width (-)=w453, precision (6)=w453) -> (F-format string=w459:string)  [unwired: 1 in]
        n234 = Number To Fractional String(number=w451, width (-)=w453, precision (6)=w453) -> (F-format string=w458:string)  [unwired: 1 in]
        n235 = Number To Fractional String(number=w450, width (-)=w453, precision (6)=w453) -> (F-format string=w457:string)  [unwired: 1 in]
        n236 = Number To Fractional String(number=w449, width (-)=w453, precision (6)=w453) -> (F-format string=w435:string)  [unwired: 1 in]
        n237 = Number To Fractional String(number=w448, width (-)=w453, precision (6)=w453) -> (F-format string=w434:string)  [unwired: 1 in]
        n238 = Number To Fractional String(number=w447, width (-)=w453, precision (6)=w453) -> (F-format string=w433:string)  [unwired: 1 in]
        n239 = Number To Fractional String(number=w446, width (-)=w453, precision (6)=w453) -> (F-format string=w432:string)  [unwired: 1 in]
        n240 = Number To Fractional String(number=w445, width (-)=w452, precision (6)=w452) -> (F-format string=w431:string)  [unwired: 1 in]
        n241 = Number To Fractional String(number=w444, width (-)=w452, precision (6)=w452) -> (F-format string=w430:string)  [unwired: 1 in]
        n242 = Number To Fractional String(number=w443, width (-)=w452, precision (6)=w452) -> (F-format string=w429:string)  [unwired: 1 in]
        n243 = Number To Fractional String(number=w442, width (-)=w452, precision (6)=w452) -> (F-format string=w428:string)  [unwired: 1 in]
        n244 = Number To Fractional String(number=w441, width (-)=w452, precision (6)=w452) -> (F-format string=w427:string)  [unwired: 1 in]
        n245 = Number To Fractional String(number=w440, width (-)=w452, precision (6)=w452) -> (F-format string=w426:string)  [unwired: 1 in]
        n246 = Number To Fractional String(number=w439, width (-)=w452, precision (6)=w452) -> (F-format string=w425:string)  [unwired: 1 in]
        n247 = Number To Fractional String(number=w438, width (-)=w452, precision (6)=w452) -> (F-format string=w424:string)  [unwired: 1 in]
        n248 = Number To Fractional String(number=w437, width (-)=w452, precision (6)=w452) -> (F-format string=w423:string)  [unwired: 1 in]
        n249 = local read "VG_RSTH"() -> (w420:bool)
        n250 = local read "VDD33A"() -> (w413:bool)
        n251 = local read "VGRSTL"() -> (w418:bool)
        n252 = local read "VDDPIX"() -> (w412:bool)
        n253 = local read "VDDCL"() -> (w416:bool)
        n254 = local read "VDDIO"() -> (w417:bool)
        n255 = local read "VDD13"() -> (w414:bool)
        n256 = local read "VTXH"() -> (w419:bool)
        n257 = local read "VTXL"() -> (w415:bool)
        n258 = Compound Arithmetic op=OR(w420, w419, w418, w417, w416, w415, w414, w413, w412) -> (w456:bool)
        n259 = Select(t="!!!", s=w456, f="") -> (s? t:f=w422:string)
        n260 = Concatenate Strings(w462, w436, w461, w436, w460, w436, w459, w436, w458, w436, w457, w436, w435, w436, w434, w436, w433, w436, w432, w436, w431, w436, w430, w436, w429, w436, w428, w436, w427, w436, w426, w436, w425, w436, w424, w436, w423, w436, w422, "\r\n") -> (w466:string)
        n261 = Format Into String(initial string=w465, w466) -> (resulting string=w454:refnum<file>)  [unwired: 2 in, 1 out]
      }
      frame #2 {
        n262 = local read "VG_RSTH"() -> (w480:bool)
        n263 = local read "Питание"() -> (w483:bool)
        n264 = local read "VDD33A"() -> (w473:bool)
        n265 = local read "VGRSTL"() -> (w478:bool)
        n266 = local read "VDDPIX"() -> (w472:bool)
        n267 = local read "VDDCL"() -> (w476:bool)
        n268 = local read "VDDIO"() -> (w477:bool)
        n269 = local read "VDD13"() -> (w474:bool)
        n270 = local read "VTXH"() -> (w479:bool)
        n271 = local read "VTXL"() -> (w475:bool)
        n272 = Compound Arithmetic op=OR(w480, w479, w478, w477, w476, w475, w474, w473, w472, "SIM_SEL") -> (w481:bool)
        "SEL" <- w481
        n273 = case shown="True" w481 {
          tunnel: [w487 w495] -> w485
          tunnel: w484 -> [w486 w494]
          tunnel: w483 -> [_ w491]
          tunnel: [w486 w490] -> w482
          frame False {
            n274 = local read "Стоп"() -> (w487:bool)
          }
          frame True {
            n275 = flat-sequence {
              tunnel: w494 -> [w499]
              tunnel: [w497] -> w492
              tunnel: w491 -> [w497]
              tunnel: [w496] -> w488
              tunnel: [w502] -> w493
              tunnel: w492 -> [w502]
              tunnel: [w501] -> w489
              tunnel: w488 -> [w501]
              tunnel: [w506] -> w495
              tunnel: w493 -> [w505]
              tunnel: [w504] -> w490
              tunnel: w489 -> [w504]
              frame #0 {
                n276 = local write "Питание"(FALSE ("Питание")) -> ()
                n277 = xnode "Read/Write Control"("FPGA VI Reference In"=w499, "Автомат"=FALSE ("Линейки")) -> ("FPGA VI Reference Out"=w496:refnum<k20>)  [unwired: 1 in, 1 out]
              }
              frame #1 {
                n278 = Wait (ms)(milliseconds to wait="SEL_Time, ms") -> ()  [unwired: 1 out]
              }
              frame #2 {
                n279 = local write "Питание"(w505) -> ()
                n280 = local read "Стоп"() -> (w506:bool)
              }
            }
          }
        }
      }
    }
    n281 = Wait (ms)(milliseconds to wait=u32 1) -> ()  [unwired: 1 out]
  }
  n282 = call <instrlib>:"niDCPower Close.vi"("instrument handle"=w6) -> ()  [unwired: 10 in, 1 out]
  n283 = call <instrlib>:"niDCPower Close.vi"("instrument handle"=w5) -> ()  [unwired: 10 in, 1 out]
  n284 = call <instrlib>:"niDCPower Close.vi"("instrument handle"=w4) -> ()  [unwired: 10 in, 1 out]
  n285 = call <instrlib>:"niDCPower Close.vi"("instrument handle"=w7) -> ()  [unwired: 10 in, 1 out]
  n286 = Close File(refnum=w15) -> ()  [unwired: 1 in, 2 out]
  n287 = xnode "Close FPGA VI Reference"("FPGA VI Reference In"=w14) -> ()  [unwired: 1 in, 1 out]
